vi "Set PID Control.vi"(8 "error in":errorcluster, 10 "Ctl Vals":cluster{"P":dbl, "I":dbl, "D":dbl}, 11 "TE Cooler in":refnum<class "TE Cooler.lvclass">) -> (0 "error out":errorcluster, 3 "TE Cooler out":refnum<class "TE Cooler.lvclass">)   [LabVIEW 2015, in "TE Cooler.lvlib" / "TE Cooler.lvclass"]
doc: "Set the control type to PID. The controller will control power the cooler adjusting for the given PID parameters entered."
uses:
  TE Cooler.lvclass
  Controls/Command.ctl
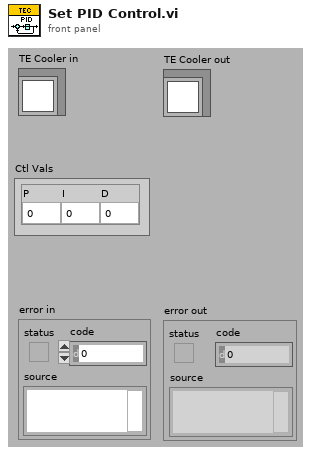
[diagram p1: front panel]
types:
  T1 = typedef "TE Cooler.lvlib/TE Cooler.lvclass/Command.ctl" = enum16{"INPUT1", "DESIRED CONTROL VALUE", "POWER OUTPUT", "ALARM STATUS", "INPUT 2", "OUTPUT CURRENT COUNTS", "ALARM TYPE", "SET TYPE DEFINE", "SENSOR TYPE", "CONTROL TYPE", "CONTROL OUTPUT POLARITY", "POWER ON/OFF", "OUTPUT SHUTDOWN IF ALARM", "FIXED DESIRED CONTROL SETTING", "PROPORTIONAL BANDWIDTH", "INTEGRAL GAIN", "DERIVATIVE GAIN", "LOW EXTERNAL SET RANGE", "HIGH EXTERNAL SET RANGE", "ALARM DEADBAND", "HIGH ALARM SETTING", "LOW ALARM SETTING", "CONTROL DEADBAND SETTING", "INPUT1 OFFSET", "INPUT2 OFFSET", "HEAT MULTIPLIER", "COOL MULTIPLIER", "OVER CURRENT COUNT COMPARE VALUE", "ALARM LATCH ENABLE", "NOT USED", "ALARM LATCH RESET", "CHOOSE SENSOR FOR ALARM FUNCTION", "CHOOSE TEMPERATURE WORKING UNITS", "EEPROM WRITE ENABLE", "OVER CURRENT CONTINUOUS", "OVER CURRENT RESTART ATTEMPTS", "JP3 DISPLAY ENABLE"}
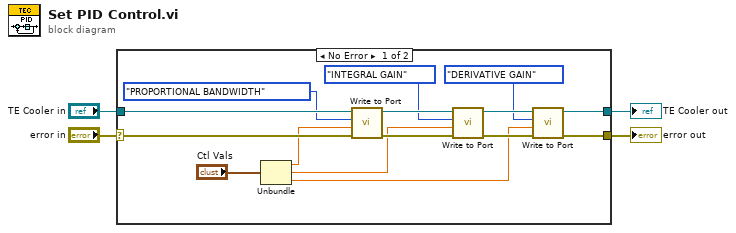
[diagram p0: block diagram]
diagram:
  n1 = case shown="No Error" "error in" {
    selector: "error in" -> [w19 w21]
    tunnel: [w11 w21] -> w3
    tunnel: [w12 w20] -> w1
    tunnel: "TE Cooler in" -> [w18 w20]
    frame No Error {
      n2 = Unbundle("Ctl Vals") -> ("P"=w7:dbl, "I"=w6:dbl, "D"=w5:dbl)
      n3 = call "Write to Port.vi"("error in"=w19, "Input Value"=w7, "TEC Cmd"=Command."PROPORTIONAL BANDWIDTH", "TE Cooler in"=w18) -> ("error out"=w9:errorcluster, "TE Cooler out"=w16:refnum<class "TE Cooler.lvclass">)  [unwired: 5 in, 1 out]
      n4 = call "Write to Port.vi"("error in"=w9, "Input Value"=w6, "TEC Cmd"=Command."INTEGRAL GAIN", "TE Cooler in"=w16) -> ("error out"=w10:errorcluster, "TE Cooler out"=w15:refnum<class "TE Cooler.lvclass">)  [unwired: 5 in, 1 out]
      n5 = call "Write to Port.vi"("error in"=w10, "Input Value"=w5, "TEC Cmd"=Command."DERIVATIVE GAIN", "TE Cooler in"=w15) -> ("error out"=w11:errorcluster, "TE Cooler out"=w12:refnum<class "TE Cooler.lvclass">)  [unwired: 5 in, 1 out]
    }
    frame Error {
    }
  }
  "error out" <- w3
  "TE Cooler out" <- w1
